vi "test Get-Set-Get Label Properties.vi"(8 "error in":errorcluster, 11 "TestCase in":refnum<class "Scripting.lvclass">) -> (0 "error out":errorcluster, 3 "TestCase out":refnum<class "Scripting.lvclass">)   [LabVIEW 2020, in "Scripting.lvclass"]
uses:
  Scripting.lvclass
  Shared/Label Properties.ctl
  Scripting.lvclass/Scripting.ctl
  <vilib>/addons/_JKI Toolkits/VI Tester/TestCase.llb/TestCase.lvclass
  Scripting/Ballard ARINC 429 Scripting.lvlib
  C:/Program Files (x86)/National Instruments/LabVIEW 2020/vi.lib/addons/_JKI Toolkits/VI Tester/TestCase.llb/TestCase.lvclass
  C:/Git/niveristand-ballard-arinc429-custom-device/Source/Custom Device Support/Tests/Unit/Scripting/Scripting.lvclass
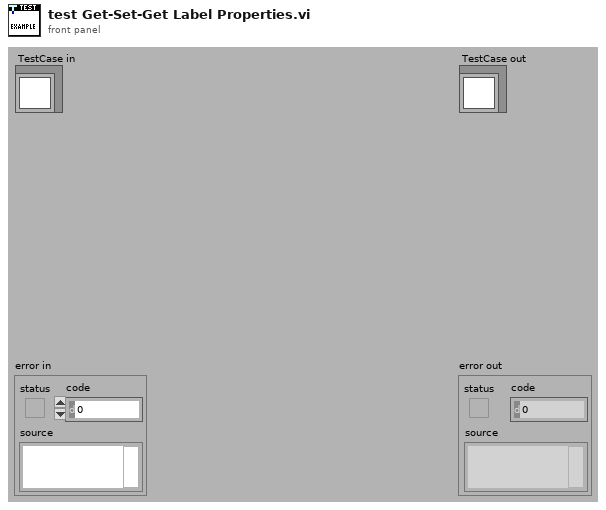
[diagram p1: front panel]
types:
  T1 = typedef "Label Properties.ctl" = cluster{"label (Dec)":i32, "SDI value":u8, "SDI enabled":bool}
  T2 = typedef "Custom Device API.lvlib/Custom Device Item Ref.ctl" = u64
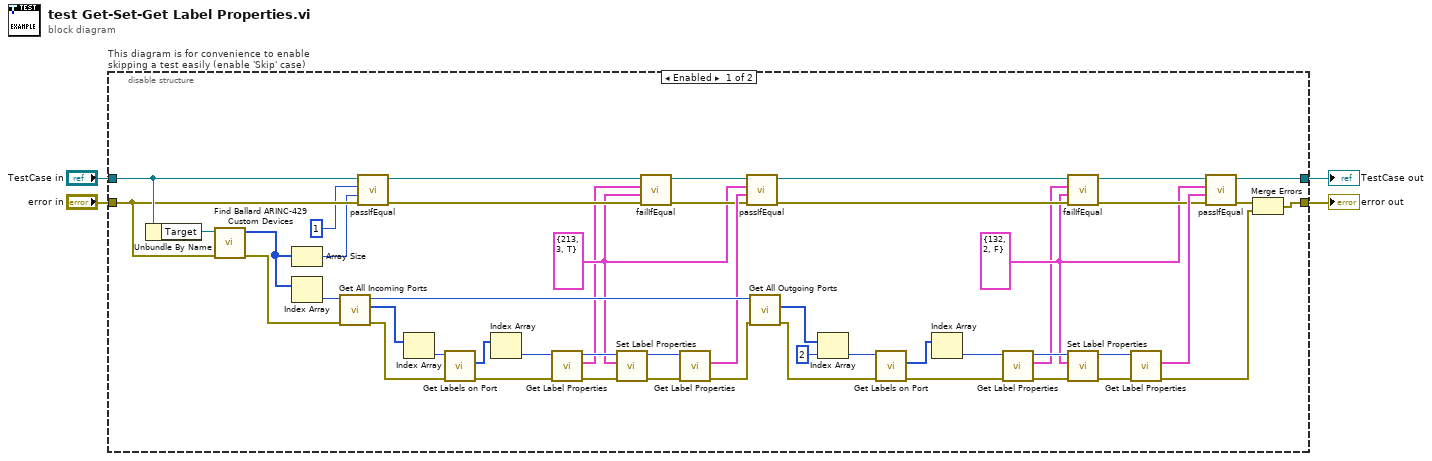
[diagram p0: block diagram]
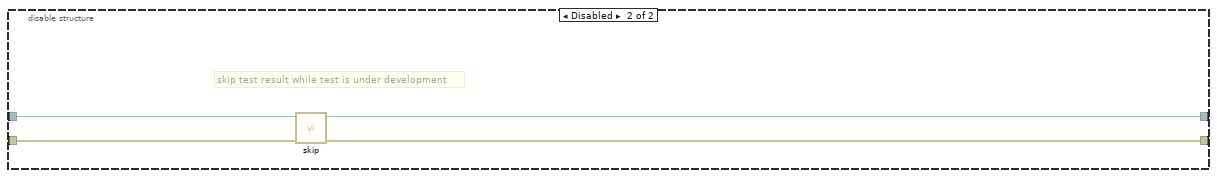
[diagram p2: hidden frame]
diagram:
  n1 = disable-structure "This diagram is for convenience to enable skipping a test easily (enable 'Skip' case)" shown="Enabled" {
    disable-tunnel: "TestCase in" -> [w51 w57]
    disable-tunnel: [w33 w55] -> w1
    disable-tunnel: [w41 w56] -> w3
    disable-tunnel: "error in" -> [w50 w54]
    frame Enabled {
      w6 = T1 {"label (Dec)"=132, "SDI value"=2, "SDI enabled"=FALSE} ("label properties")
      w12 = T1 {"label (Dec)"=213, "SDI value"=3, "SDI enabled"=TRUE} ("label properties")
      n2 = Unbundle By Name(w51) -> ("Target"=w53:refnum<k24>)
      n3 = call "Find Ballard ARINC-429 Custom Devices.vi"("error in"=w50, "target"=w53) -> ("error out"=w45:errorcluster, "Ballard ARINC-429 custom devices"=w49:u64[])  [unwired: 8 in]
      n4 = Array Size(array=w49) -> (size(s)=w47:i32)
      n5 = Index Array(array=w49) -> (element=w52:u64)  [unwired: 1 in]
      n6 = call "Get All Incoming Ports.vi"("error in"=w45, "Ballard ARINC 429 ref"=w52) -> ("error out"=w39:errorcluster, "Port refs"=w46:T2[], "Ballard ARINC 429 ref out"=w44:T2)  [unwired: 7 in]
      n7 = call-dynamic "passIfEqual.vi"("error in (no error)"=w50, "y"=w47, "x"=1 ("size(s)"), "TestCase in"=w51) -> ("error out"=w15:errorcluster, "TestCase out"=w16:refnum<class "Scripting.lvclass">)  [unwired: 6 in]
      n8 = Index Array(array=w46) -> (element=w40:T2)  [unwired: 1 in]
      n9 = call "Get Labels on Port.vi"("error in"=w39, "port ref"=w40) -> ("error out"=w27:errorcluster, "label references"=w35:T2[])  [unwired: 6 in, 2 out]
      n10 = Index Array(array=w35) -> (element=w28:T2)  [unwired: 1 in]
      n11 = call "Get Label Properties.vi"("error in"=w27, "label ref in"=w28) -> ("error out"=w31:errorcluster, "label properties"=w11:T1, "label ref out"=w32:T2)  [unwired: 7 in]
      n12 = call "Set Label Properties.vi"("error in"=w31, "label properties"=w12, "label ref"=w32) -> ("error out"=w29:errorcluster, "label ref out"=w30:T2)  [unwired: 7 in]
      n13 = call-dynamic "failIfEqual.vi"("error in (no error)"=w15, "y"=w12, "x"=w11, "TestCase in"=w16) -> ("error out"=w13:errorcluster, "TestCase out"=w14:refnum<class "Scripting.lvclass">)  [unwired: 6 in]
      n14 = call "Get Label Properties.vi"("error in"=w29, "label ref in"=w30) -> ("error out"=w26:errorcluster, "label properties"=w25:T1)  [unwired: 7 in, 1 out]
      n15 = call-dynamic "passIfEqual.vi"("error in (no error)"=w13, "y"=w25, "x"=w12, "TestCase in"=w14) -> ("error out"=w9:errorcluster, "TestCase out"=w10:refnum<class "Scripting.lvclass">)  [unwired: 6 in]
      n16 = call "Get All Outgoing Ports.vi"("error in"=w26, "Ballard ARINC 429 ref"=w44) -> ("error out"=w38:errorcluster, "Port refs"=w43:T2[])  [unwired: 7 in, 1 out]
      n17 = Index Array(array=w43, index=2) -> (element=w37:T2)
      n18 = call "Get Labels on Port.vi"("error in"=w38, "port ref"=w37) -> ("error out"=w19:errorcluster, "label references"=w36:T2[])  [unwired: 6 in, 2 out]
      n19 = Index Array(array=w36) -> (element=w20:T2)  [unwired: 1 in]
      n20 = call "Get Label Properties.vi"("error in"=w19, "label ref in"=w20) -> ("error out"=w22:errorcluster, "label properties"=w5:T1, "label ref out"=w21:T2)  [unwired: 7 in]
      n21 = call-dynamic "failIfEqual.vi"("error in (no error)"=w9, "y"=w6, "x"=w5, "TestCase in"=w10) -> ("error out"=w7:errorcluster, "TestCase out"=w8:refnum<class "Scripting.lvclass">)  [unwired: 6 in]
      n22 = call "Set Label Properties.vi"("error in"=w22, "label properties"=w6, "label ref"=w21) -> ("error out"=w24:errorcluster, "label ref out"=w23:T2)  [unwired: 7 in]
      n23 = call "Get Label Properties.vi"("error in"=w24, "label ref in"=w23) -> ("error out"=w18:errorcluster, "label properties"=w17:T1)  [unwired: 7 in, 1 out]
      n24 = call-dynamic "passIfEqual.vi"("error in (no error)"=w7, "y"=w17, "x"=w6, "TestCase in"=w8) -> ("error out"=w34:errorcluster, "TestCase out"=w33:refnum<class "Scripting.lvclass">)  [unwired: 6 in]
      n25 = Merge Errors(w34, w18) -> (w41:errorcluster)
    }
    frame Disabled {
      # "skip test result while test is under development"
      n26 = call <vilib>:"skip.vi"("error in (no error)"=w54, "TestCase in"=w57) -> ("error out"=w56:errorcluster, "TestCase out"=w55:refnum<class "Scripting.lvclass">)  [unwired: 8 in]
    }
  }
  "error out" <- w3
  "TestCase out" <- w1
